vi "Read Continuous flag.vi"(8 "error in (no error)":errorcluster, 11 "Schedule in":refnum<class "Schedule.lvclass">) -> (0 "error out":errorcluster, 2 "Continuous flag":bool, 3 "Schedule out":refnum<class "Schedule.lvclass">)   [LabVIEW 2020, in "TALOS.lvlib" / "Run Utilities.lvlib" / "Schedule.lvclass"]
doc: "Get value of Continuous Flag (is this schedule supposed to be running continuously)"
uses:
  Schedule.lvclass
  Schedule.lvclass/Schedule.ctl
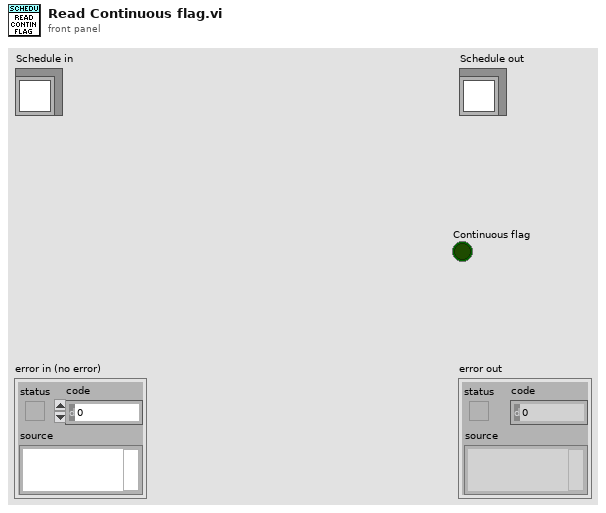
[diagram p1: front panel]
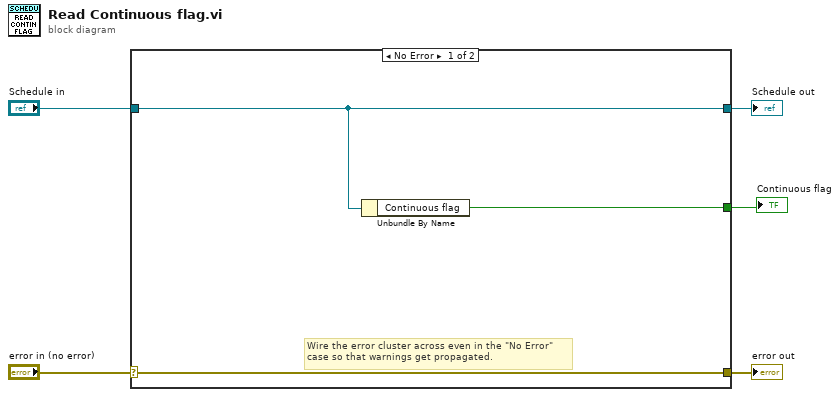
[diagram p0: block diagram]
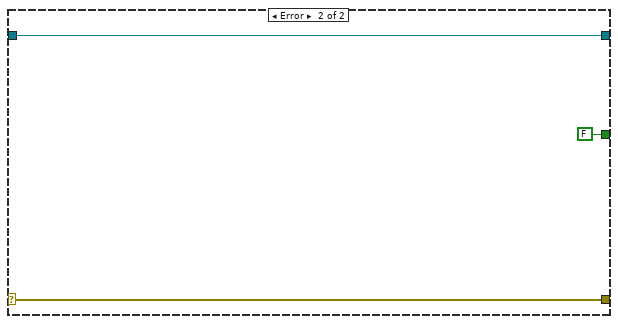
[diagram p2: hidden frame]
diagram:
  n1 = case shown="No Error" "error in (no error)" {
    selector: "error in (no error)" -> [w8 w11]
    tunnel: [w8 w11] -> w4
    tunnel: [w7 w10] -> w2
    tunnel: "Schedule in" -> [w7 w10]
    tunnel: [w6 FALSE ("Continuous flag")] -> w1
    frame No Error {
      # "Wire the error cluster across even in the \"No Error\"\ncase so that warnings get propagated."
      n2 = Unbundle By Name(w7) -> ("Continuous flag"=w6:bool)
    }
    frame Error {
    }
  }
  "error out" <- w4
  "Schedule out" <- w2
  "Continuous flag" <- w1
